vi "Variant to 2D Array.vi"(2 "error in (no error)":errorcluster, 3 "Value":variant) -> (0 "error out":errorcluster, 1 "Array":dbl[][](array[numeric]))   [LabVIEW 2019, in "graph_utilities.lvclass"]
uses:
  graph_utilities.lvclass
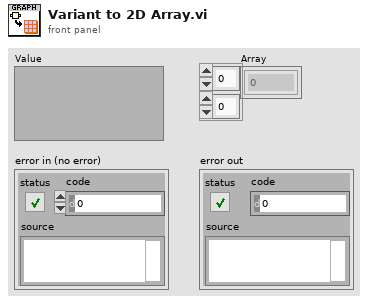
[diagram p1: front panel]
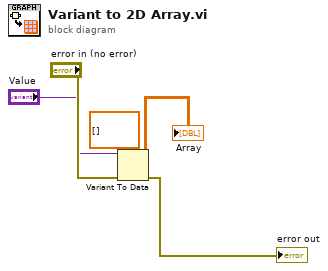
[diagram p0: block diagram]
diagram:
  n1 = Variant To Data(error in="error in (no error)", type=dbl[][] [], Variant="Value") -> (data=→"Array":dbl[][], error out=→"error out":errorcluster)
